vi "New RTTarget.vi"(8 "instVIpath":path, 9 "target location":string, 11 "RTTarget in":refnum<class "RTTarget.lvclass">) -> (3 "RTTarget out":refnum<class "RTTarget.lvclass">)   [LabVIEW 2020, in "NI_TargetHelper.lvlib" / "RTTarget.lvclass"]
uses:
  <vilib>/TargetSupport/NI_TargetHelper/RTTarget/RTTarget.lvclass
  <vilib>/TargetSupport/NI_TargetHelper/RTTarget/RTTarget.lvclass/RTTarget.ctl
  <vilib>/TargetSupport/NI_TargetHelper/NI_TargetHelper.lvlib
panel:
  out "error out":errorcluster
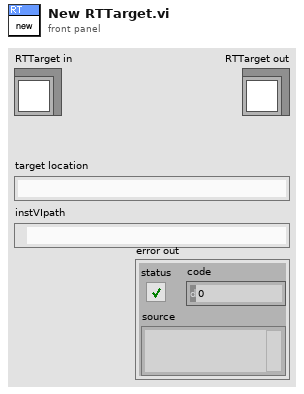
[diagram p1: front panel]
types:
  T1 = typedef "NI_TargetHelper.lvlib/Instance VIref.ctl" = refnum<vi>
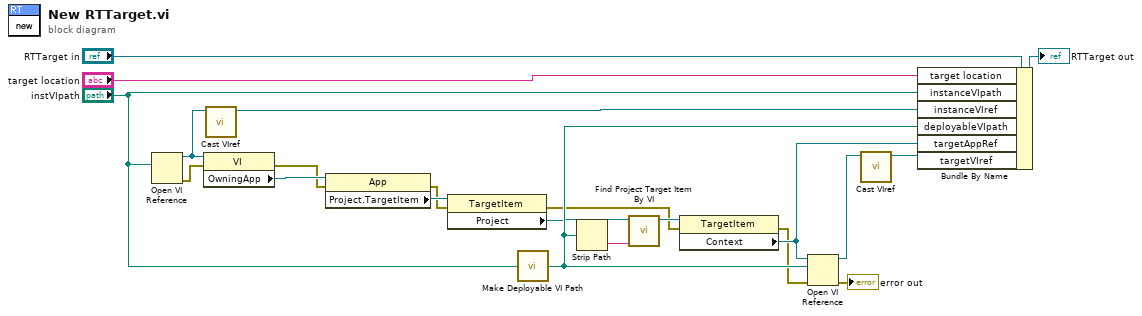
[diagram p0: block diagram]
diagram:
  n1 = Open VI Reference(vi path="instVIpath") -> (vi reference=w1:refnum<vi>, error out=w8:errorcluster)  [unwired: 5 in]
  n2 = property class="VI"(reference=w1, error in=w8) -> (error out=w7:errorcluster, "OwningApp"=w14:refnum<vi>)  [unwired: 1 out]
  n3 = call <vilib>:"Cast VIref.vi"("VI Refnum"=w1) -> ("instVIref"=w2:T1)  [unwired: 10 in]
  n4 = property class="App"(reference=w14, error in=w7) -> (error out=w6:errorcluster, "Project.TargetItem"=w15:refnum<vi>)  [unwired: 1 out]
  n5 = property class="TargetItem"(reference=w15, error in=w6) -> (error out=w5:errorcluster, "Project"=w13:refnum<vi>)  [unwired: 1 out]
  n6 = call <vilib>:"Make Deployable VI Path.vi"("instance path"="instVIpath") -> ("deployable path"=w17:path)
  n7 = Strip Path(path=w17) -> (name=w16:string)  [unwired: 1 out]
  n8 = call <vilib>:"Find Project Target Item By VI.vi"("vi name"=w16, "project"=w13) -> ("TargetItem Refnum"=w12:refnum<vi>)  [unwired: 8 in, 1 out]
  n9 = property class="TargetItem"(reference=w12, error in=w5) -> (error out=w4:errorcluster, "Context"=w11:refnum<vi>)  [unwired: 1 out]
  n10 = Open VI Reference(application reference (local)=w11, vi path=w17, error in (no error)=w4) -> (vi reference=w10:refnum<vi>, error out=→"error out":errorcluster)  [unwired: 3 in]
  n11 = call <vilib>:"Cast VIref.vi"("VI Refnum"=w10) -> ("instVIref"=w9:T1)  [unwired: 10 in]
  n12 = Bundle By Name(cluster="RTTarget in", "target location"="target location", "instanceVIpath"="instVIpath", "instanceVIref"=w2, "deployableVIpath"=w17, "targetAppRef"=w11, "targetVIref"=w9) -> (→"RTTarget out":refnum<class "RTTarget.lvclass">)
